vi "WPI_CameraIsCameraRefUSBAddress.vi"(8 "error in (no error)":errorcluster, 10 "Enumerate":bool, 11 "CameraDevRef":T1) -> (0 "error out":errorcluster, 1 "USB?":bool, 2 "Camera Address Out":string, 3 "CameraDevRef out":T1)   [LabVIEW 2017]
doc: "A wrapper around the USB Address function. This function determines if a DevRef references a USB camera, and resolves it if it is.\n\nThis software is licensed. Open the labview\\readme\\WPI Robotics Library Open Source License.txt file for more information."
uses:
  <vilib>/Rock Robotics/WPI/Camera/WPI_CameraDevRef.ctl
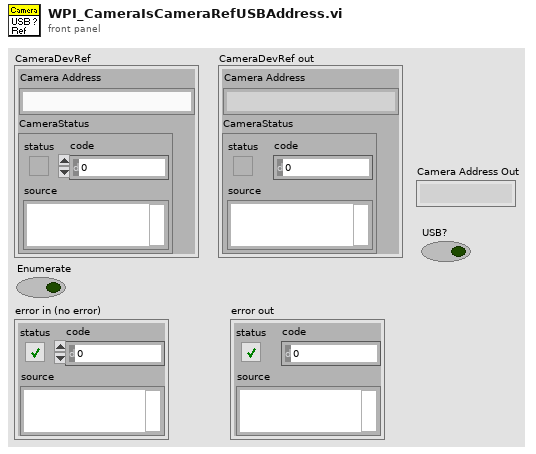
[diagram p1: front panel]
types:
  T1 = typedef "WPI_CameraDevRef.ctl" = cluster{"Camera Address":string, "CameraStatus":errorcluster}
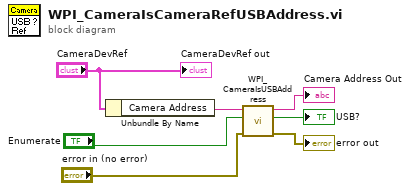
[diagram p0: block diagram]
diagram:
  n1 = Unbundle By Name("CameraDevRef") -> ("Camera Address"=w3:string)
  n2 = call <vilib>:"WPI_CameraIsUSBAddress.vi"("error in (no error)"="error in (no error)", "Enumerate?"="Enumerate", "Camera Address In"=w3) -> ("error out"=→"error out":errorcluster, "USB?"=→"USB?":bool, "Camera Address Out"=→"Camera Address Out":string)  [unwired: 6 in]
  "CameraDevRef out" <- "CameraDevRef"
